vi "Intan_saveHeaderInfo.vi"(3 "error in":errorcluster, 4 "header text":string, 5 "DataFilePath":path=path "C:/write-read example.txt") -> (0 "error out":errorcluster, 1 "hdr_file_ref_num_out":refnum<file>, 2 "HeaderFilePath":path)   [LabVIEW 2017]
doc: "Saves to header text file Intan config results, specifying frequency, hardware filters selected, etc. A date and time stamp is appended just prior to writing. This is done to ensure that the timestamp corresoponds as closely as possible to the time at which the data stream begins."
panel:
  out "date_and_time_string":string
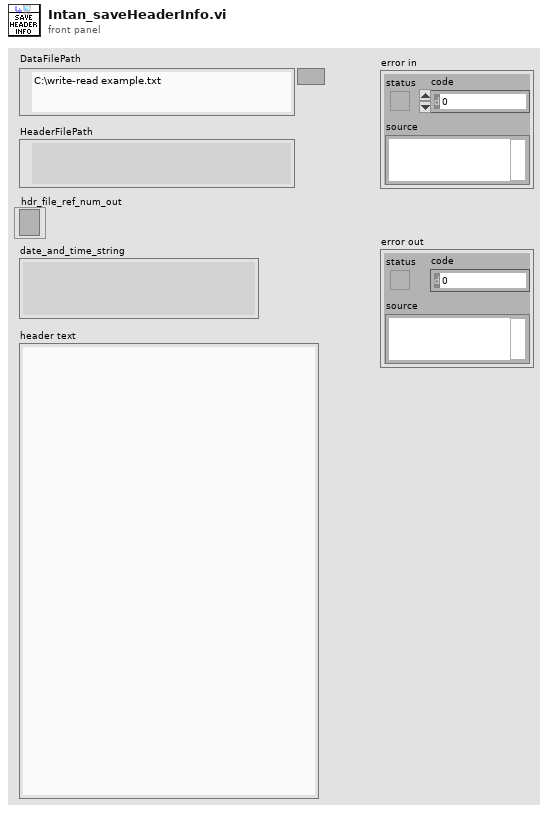
[diagram p1: front panel]
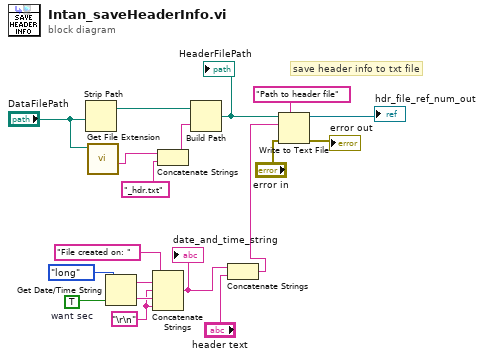
[diagram p0: block diagram]
diagram:
  w7 = "\r\n"
  w13 = TRUE  # want sec
  # "save header info to txt file"
  n1 = Strip Path(path="DataFilePath") -> (stripped path=w15:path)  [unwired: 1 out]
  n2 = call <vilib>:"Get File Extension.vi"("file"="DataFilePath") -> ("filename without extension"=w3:string)  [unwired: 6 in, 4 out]
  n3 = Get Date/Time String(date format (0)=enum16{"short", "long", "abbreviated"}."long", want seconds? (F)=w13) -> (date string=w14:string, time string=w8:string)  [unwired: 1 in]
  n4 = Concatenate Strings("File created on: " ("string"), w14, w7, w8, w7) -> (w12:string)
  "date_and_time_string" <- w12
  n5 = Concatenate Strings(w3, "_hdr.txt" ("name or relative path")) -> (w5:string)
  n6 = Build Path(base path=w15, name or relative path=w5) -> (appended path=w18:path)
  "HeaderFilePath" <- w18
  n7 = Concatenate Strings(w12, "header text") -> (w10:string)
  n8 = Write to Text File(prompt (Choose or enter file path)="Path to header file", file (use dialog)=w18, text=w10, error in="error in") -> (refnum out=→"hdr_file_ref_num_out":refnum<file>, error out=→"error out":errorcluster)  [unwired: 1 out]
